vi "Get NIST Info.vi"(3 "error in (no error)":errorcluster, 4 "timeout ms (60000)":i32=60000, 5 "NTP port":u16=13, 6 "time server":T1(ring)) -> (0 "error out":errorcluster, 1 "time":cluster{i32, i32, i32}, 2 "date":cluster{i32, i32, i32})   [LabVIEW 2012]
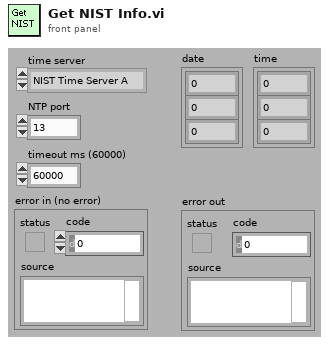
[diagram p1: front panel]
types:
  T1 = enum16{"NIST Time Server A", "NIST Time Server B"}
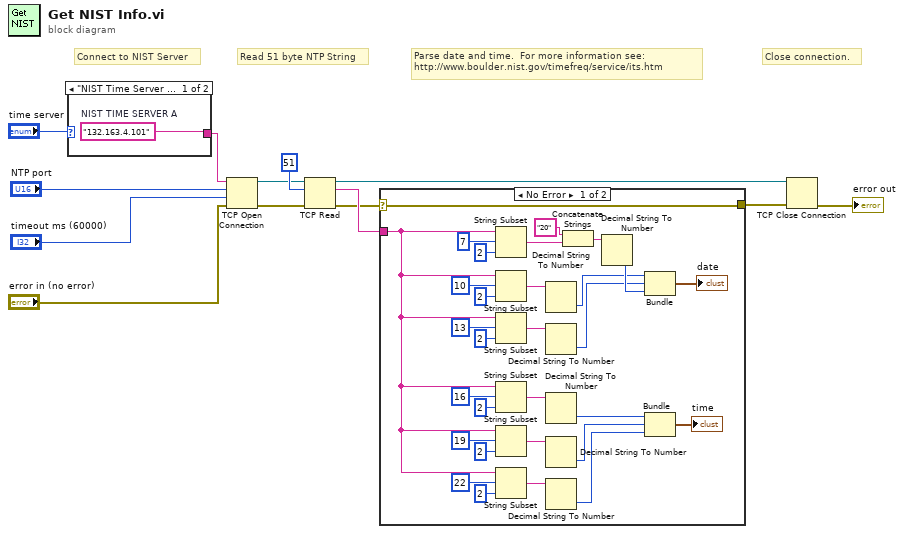
[diagram p0: block diagram]
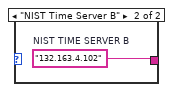
[diagram p3: hidden frame]
diagram:
  # "Close connection."
  # "Parse date and time.  For more information see:\nhttp://www.boulder.nist.gov/timefreq/service/its.htm"
  # "Connect to NIST Server"
  # "Read 51 byte NTP String"
  n1 = case shown="\"NIST Time Server A\", Default" "time server" {
    tunnel: [w14 w15] -> w10
    frame "NIST Time Server A", Default {
      w14 = "132.163.4.101"  # NIST TIME SERVER A
    }
    frame "NIST Time Server B" {
      w15 = "132.163.4.102"  # NIST TIME SERVER B
    }
  }
  n2 = TCP Open Connection(address=w10, remote port or service name="NTP port", timeout ms (60000)="timeout ms (60000)", error in (no error)="error in (no error)") -> (connection ID=w11:refnum<k5>, error out=w8:errorcluster)  [unwired: 1 in]
  n3 = TCP Read(connection ID=w11, bytes to read=51, error in (no error)=w8) -> (connection ID out=w9:refnum<k5>, data out=w3:string, error out=w2:errorcluster)  [unwired: 2 in]
  n4 = case shown="No Error" w2 {
    selector: w2 -> [w16 w46]
    tunnel: w3 -> [w23 _]
    tunnel: [w16 w46] -> w1
    frame No Error {
      n5 = String Subset(string=w23, offset (0)=7, length (rest)=2 ("length (rest)")) -> (substring=w43:string)
      n6 = String Subset(string=w23, offset (0)=10, length (rest)=2 ("length (rest)")) -> (substring=w35:string)
      n7 = String Subset(string=w23, offset (0)=13, length (rest)=2 ("length (rest)")) -> (substring=w36:string)
      n8 = String Subset(string=w23, offset (0)=16, length (rest)=2 ("length (rest)")) -> (substring=w22:string)
      n9 = String Subset(string=w23, offset (0)=19, length (rest)=2 ("length (rest)")) -> (substring=w31:string)
      n10 = String Subset(string=w23, offset (0)=22, length (rest)=2 ("length (rest)")) -> (substring=w30:string)
      n11 = Decimal String To Number(string=w35) -> (number=w33:i32)  [unwired: 2 in, 1 out]
      n12 = Decimal String To Number(string=w36) -> (number=w32:i32)  [unwired: 2 in, 1 out]
      n13 = Decimal String To Number(string=w22) -> (number=w21:i32)  [unwired: 2 in, 1 out]
      n14 = Decimal String To Number(string=w31) -> (number=w20:i32)  [unwired: 2 in, 1 out]
      n15 = Decimal String To Number(string=w30) -> (number=w19:i32)  [unwired: 2 in, 1 out]
      n16 = Concatenate Strings("20" ("string"), w43) -> (w37:string)
      n17 = Decimal String To Number(string=w37) -> (number=w34:i32)  [unwired: 2 in, 1 out]
      n18 = Bundle(w33, w32, w34) -> (→"date":cluster{i32, i32, i32})  [unwired: 1 in]
      n19 = Bundle(w21, w20, w19) -> (→"time":cluster{i32, i32, i32})  [unwired: 1 in]
    }
    frame Error {
    }
  }
  n20 = TCP Close Connection(connection ID=w9, error in (no error)=w1) -> (error out=→"error out":errorcluster)  [unwired: 1 in, 1 out]
